vi "ReadFromLocalFile.vi"() -> ()   [LabVIEW 2012]
uses:
  <vilib>/Analysis/NI_AALBase.lvlib
panel:
  out "Dispersioon (vasak)":dbl format="%0.2f"
  out "Standardhälve (vasak)":dbl format="%0.2f"
  out "Keskmine (vasak)":dbl format="%0.2f"
  out "Dispersioon (parem)":dbl format="%0.2f"
  out "Standardhälve (parem)":dbl format="%0.2f"
  out "Keskmine (parem)":dbl format="%0.2f"
  out "Parem":cluster{timestamp[], dbl[]}(graph)
  out "Vasak":cluster{timestamp[], dbl[]}(graph)
  in  "Faili tee":path
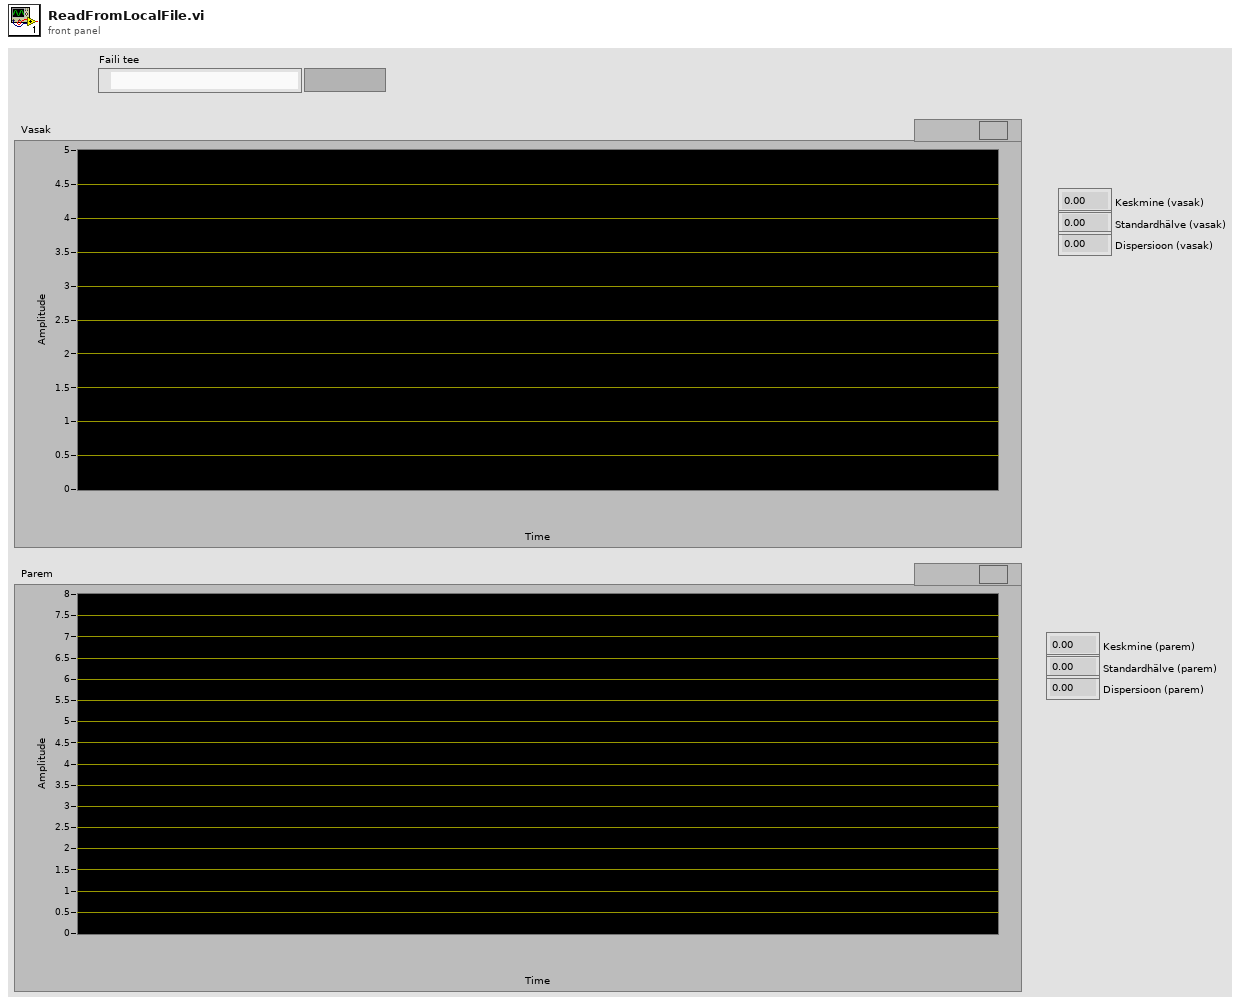
[diagram p1: front panel]
types:
  T1 = enum16{"open", "replace", "create", "open or create", "replace or create", "replace or create with confirmation"}
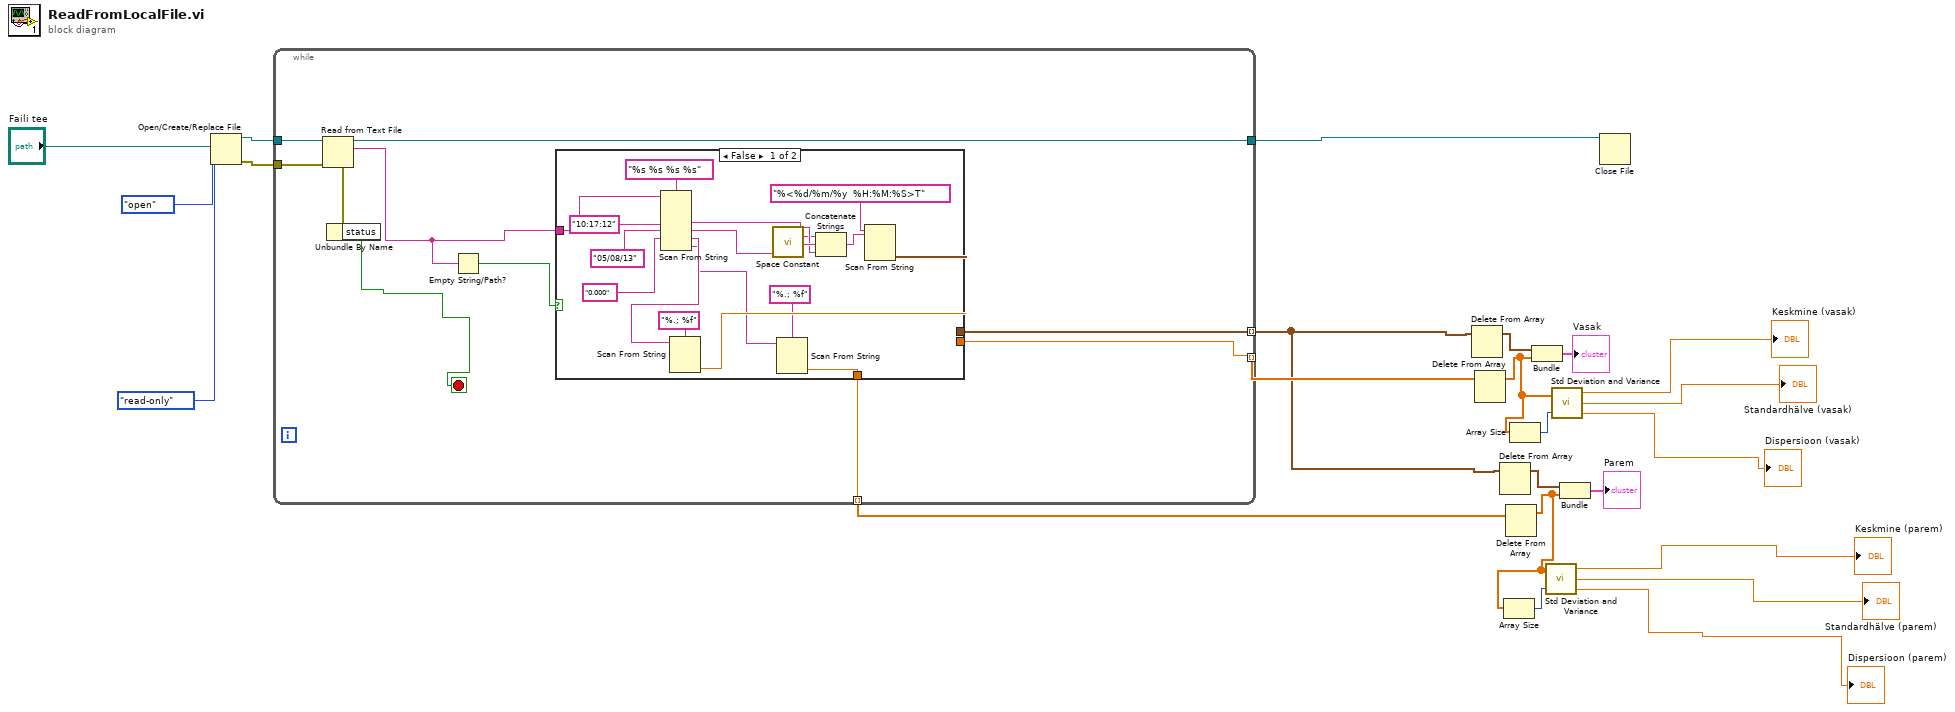
[diagram p0: block diagram]
diagram:
  n1 = Open/Create/Replace File(file path (use dialog)="Faili tee", operation (0:open)=T1."open", access (0:read/write)=enum16{"read/write", "read-only", "write-only"}."read-only") -> (refnum out=w22:refnum<file>, error out=w23:errorcluster)  [unwired: 3 in, 1 out]
  n2 = while {
    tunnel: w23 -> [w33]
    tunnel: w22 -> [w31]
    tunnel: [w30] -> w18
    tunnel: [w28] -> w16 mode=indexing
    tunnel: [w29] -> w11 mode=indexing
    tunnel: [w24] -> w12 mode=indexing
    stop <- w25 stop-if-true
    n3 = Read from Text File(file (use dialog)=w31, error in=w33) -> (refnum out=w30:refnum<file>, text=w27:string, error out=w32:errorcluster)  [unwired: 2 in, 1 out]
    n4 = Unbundle By Name(w32) -> ("status"=w25:bool)
    n5 = Empty String/Path?(string/path=w27) -> (empty?=w26:bool)
    n6 = case shown="False" w26 {
      tunnel: [w38 _] -> w29
      tunnel: [w37 _] -> w28
      tunnel: w27 -> [w39 _]
      tunnel: [w34 _] -> w24
      frame False {
        n7 = Scan From String(format string="%s %s %s %s", input string=w39, default 1="10:17:12", default 2="05/08/13", default 3="0.000") -> (output 1=w46:string, output 2=w45:string, output 3=w48:string, output 4=w35:string)  [unwired: 3 in, 3 out]
        n8 = Scan From String(format string="%.; %f", input string=w48) -> (output 1=w37:dbl)  [unwired: 3 in, 3 out]
        n9 = call <vilib>:"Space Constant.vi"() -> ("String"=w47:string)
        n10 = Scan From String(format string="%.; %f", input string=w35) -> (output 1=w34:dbl)  [unwired: 3 in, 3 out]
        n11 = Concatenate Strings(w45, w47, w46) -> (w43:string)
        n12 = Scan From String "Scan From String"(format string="%<%d/%m/%y  %H:%M:%S>T", input string=w43) -> (output 1=w38:timestamp)  [unwired: 3 in, 3 out]
      }
      frame True {
      }
    }
  }
  n13 = Delete From Array(array=w11) -> (array with subset deleted=w15:timestamp[])  [unwired: 2 in, 1 out]
  n14 = Delete From Array(array=w16) -> (array with subset deleted=w10:dbl[])  [unwired: 2 in, 1 out]
  n15 = Delete From Array(array=w11) -> (array with subset deleted=w13:timestamp[])  [unwired: 2 in, 1 out]
  n16 = Delete From Array(array=w12) -> (array with subset deleted=w7:dbl[])  [unwired: 2 in, 1 out]
  n17 = Array Size(array=w7) -> (size(s)=w8:i32)
  n18 = Array Size(array=w10) -> (size(s)=w9:i32)
  n19 = Bundle(w15, w10) -> (→"Vasak":cluster{timestamp[], dbl[]})  [unwired: 1 in]
  n20 = call <vilib>:"Std Deviation and Variance.vi"("X"=w7, "Weighting (Sample)"=w8) -> ("mean"=→"Keskmine (parem)":dbl, "standard deviation"=→"Standardhälve (parem)":dbl, "variance"=→"Dispersioon (parem)":dbl)
  n21 = call <vilib>:"Std Deviation and Variance.vi"("X"=w10, "Weighting (Sample)"=w9) -> ("mean"=→"Keskmine (vasak)":dbl, "standard deviation"=→"Standardhälve (vasak)":dbl, "variance"=→"Dispersioon (vasak)":dbl)
  n22 = Bundle(w13, w7) -> (→"Parem":cluster{timestamp[], dbl[]})  [unwired: 1 in]
  n23 = Close File(refnum=w18) -> ()  [unwired: 1 in, 2 out]
